vi "Test Print.vi"() -> ()   [LabVIEW 2014, in "Arduino SoftwareSerial Wrapper.lvlib"]
uses:
  Arduino SoftwareSerial Wrapper.lvlib
panel:
  out "Error Out":errorcluster
  in  "Error In":errorcluster
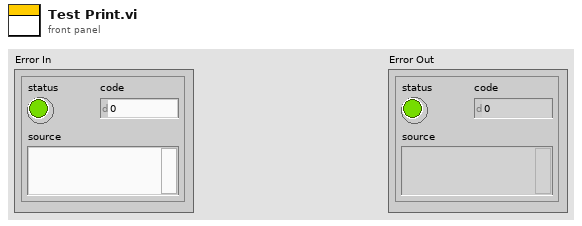
[diagram p1: front panel]
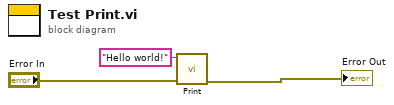
[diagram p0: block diagram]
diagram:
  n1 = call "Print.vi"("Error In"="Error In", "String to print"="Hello world!") -> ("Error Out"=→"Error Out":errorcluster)  [unwired: 9 in]
